vi "LoadPanel.vi"(0 "VI in":refnum<vi>, 5 "Panel Name":string, 11 "error in (no error)":errorcluster, 12 "milliseconds to wait":u32) -> (4 "VI out":refnum<vi>, 15 "error out":errorcluster)   [LabVIEW 2016, in "Drona Test.lvlib"]
uses:
  Drona Test.lvlib
  main/apis/Stimulus/ValueSignal/ValueSignalByPathString.vi
  main/Drona.lvlib
  main/apis/Stimulus/ValueSignal/ValueSignal.lvlib
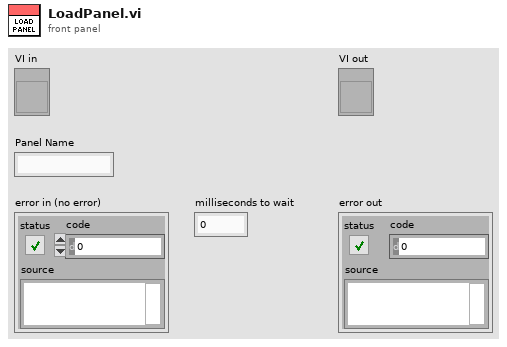
[diagram p1: front panel]
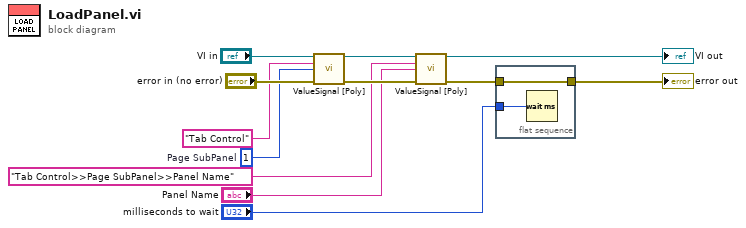
[diagram p0: block diagram]
diagram:
  w3 = 1  # Page SubPanel
  n1 = call-poly "ValueSignal [Poly].vi"("VI Reference In"="VI in", "Control Path"="Tab Control", "Value (Signaling)"=w3, "error in"="error in (no error)") -> ("VI Reference Out"=w7:refnum<vi>, "error out"=w6:errorcluster)  [unwired: 10 in]
  n2 = call-poly "ValueSignal [Poly].vi"("VI Reference In"=w7, "Control Path"="Tab Control>>Page SubPanel>>Panel Name", "Value (Signaling)"="Panel Name", "error in"=w6) -> ("VI Reference Out"=→"VI out":refnum<vi>, "error out"=w10:errorcluster)  [unwired: 10 in]
  n3 = flat-sequence {
    tunnel: [w14] -> w9
    tunnel: w10 -> [w14]
    tunnel: "milliseconds to wait" -> [w13]
    frame #0 {
      n4 = Wait (ms)(milliseconds to wait=w13) -> ()  [unwired: 1 out]
    }
  }
  "error out" <- w9
